vi "Node - Read Imported Channels.vi"(8 "error in (no error)":errorcluster, 10 "Node Name":string, 11 "Compiled.Settings In":T1) -> (0 "error out":errorcluster, 2 "Local Channels Table out":string[][](array[string]), 3 "Compiled.Settings Out":T1)   [LabVIEW 2016, in "PXImc Custom Device System Explorer.lvlib"]
uses:
  PXImc Custom Device System Explorer.lvlib
  Shared/Compiled.Settings.ctl
  <vilib>/NI Veristand/VeriStand Data/Byte Buffer/Byte Buffer.lvclass
  PXImc Router/Controls/Target Type.ctl
  PXImc Router/Controls/Router - Configuration.ctl
  PXImc Router/Controls/Router/Node Block R-W Properties.ctl
  PXImc Router/Controls/Router/Block Properties.ctl
  PXImc Router/Controls/Router/Router - PXImc Properties.ctl
  PXImc Router/Controls/Router/Router - PXImc Card Properties.ctl
  PXImc Router/Controls/Node Data.ctl
  PXImc Router/Controls/Node/Node - PXImc Parameters.ctl
  PXImc Router/Controls/Node/Node - Writer Data.ctl
  PXImc Router/Controls/Node/Node Ch Properties.ctl
  PXImc Router/Controls/Data Type.ctl
  PXImc Router/Controls/Node/Node - Readers Data.ctl
  PXImc Router/Controls/Node/Node - Reader Data.ctl
  <vilib>/Utility/file.llb/Read Delimited Spreadsheet (string).vi
  PXImc Router/PXImc Router.lvlib
  Shared/PXImc Custom Device Shared.lvlib
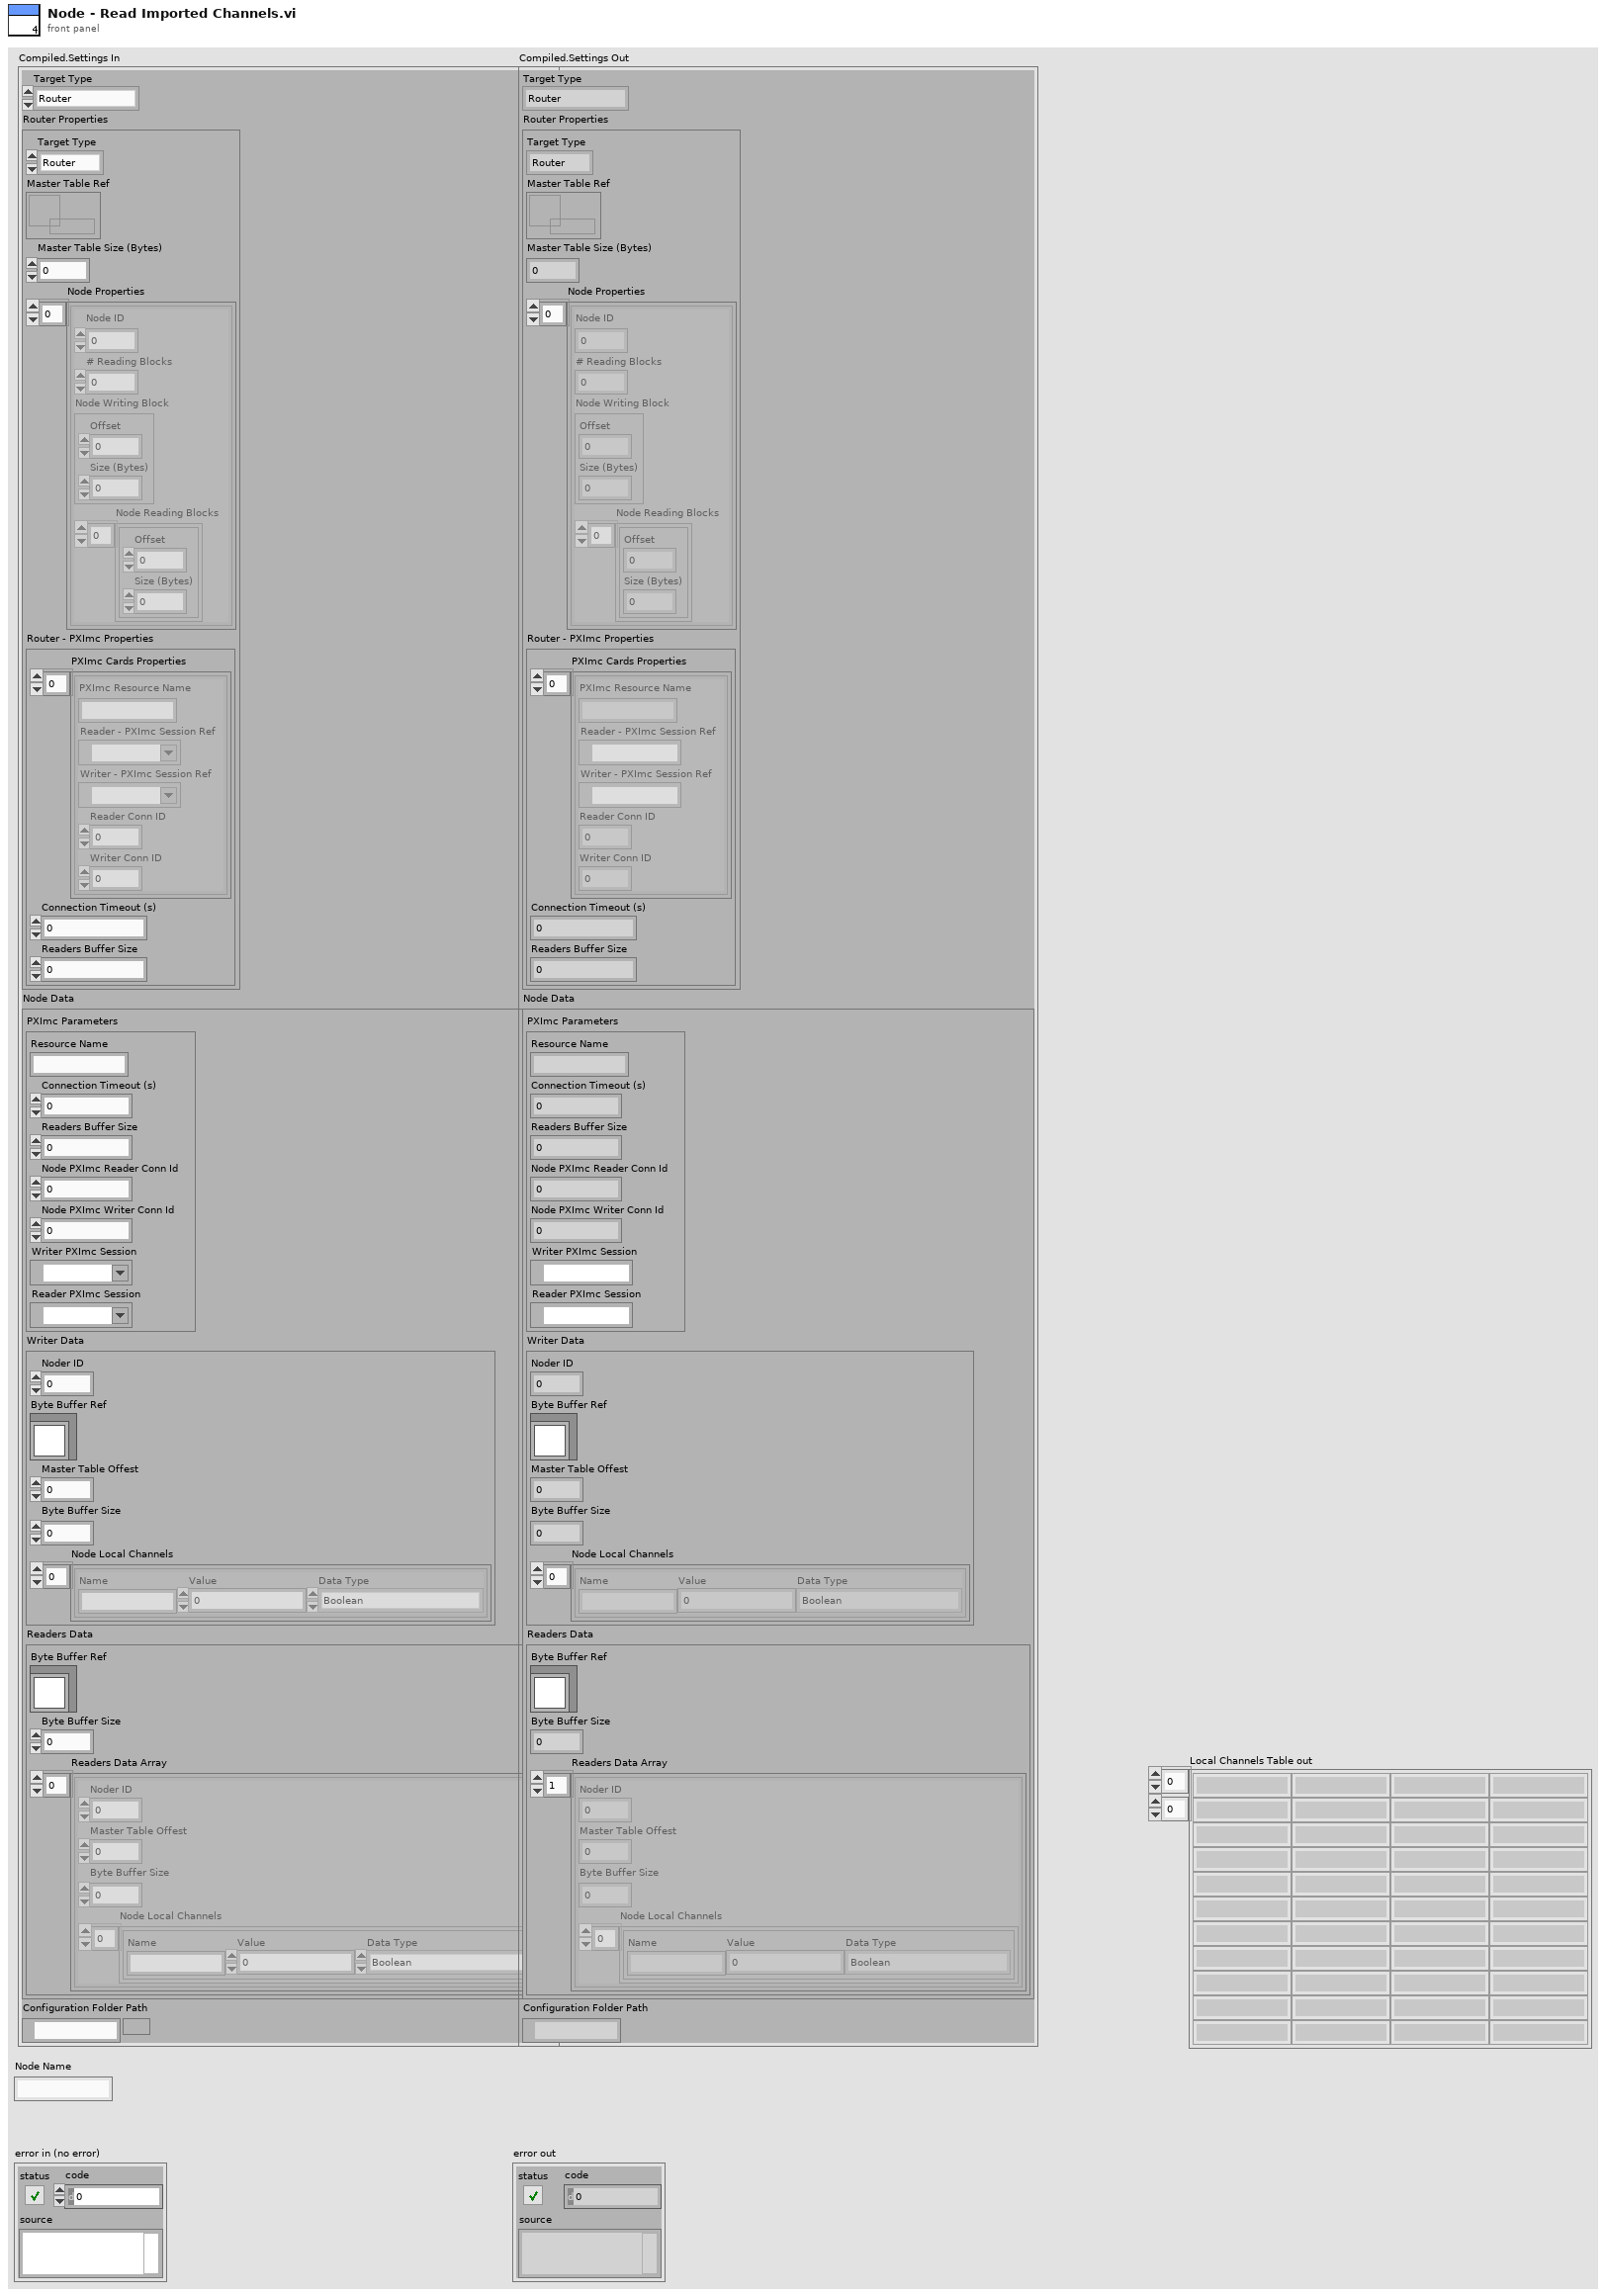
[diagram p1: front panel]
types:
  T1 = typedef "PXImc Custom Device Shared.lvlib/Compiled.Settings.ctl" = cluster{"Target Type":T2, "Router Properties":T3, "Node Data":T8, "Configuration Folder Path":path}
  T2 = typedef "PXImc Router.lvlib/Target Type.ctl" = enum16{"Router", "Node"}
  T3 = typedef "PXImc Router.lvlib/Router - Configuration.ctl" = cluster{"Target Type":T2, "Master Table Ref":refnum<data-value>, "Master Table Size (Bytes)":u32, "Node Properties":T4[], "Router - PXImc Properties":T6}
  T4 = typedef "PXImc Router.lvlib/Node Block R-W Properties.ctl" = cluster{"Node ID":u32, "# Reading Blocks":u32, "Node Writing Block":T5, "Node Reading Blocks":T5[]}
  T5 = typedef "PXImc Router.lvlib/Block Properties.ctl" = cluster{"Offset":u32, "Size (Bytes)":u32}
  T6 = typedef "PXImc Router.lvlib/Router - PXImc Properties.ctl" = cluster{"PXImc Cards Properties":T7[], "Connection Timeout (s)":dbl, "Readers Buffer Size":u64}
  T7 = typedef "PXImc Router.lvlib/Router - PXImc Card Properties.ctl" = cluster{"PXImc Resource Name":string, "Reader - PXImc Session Ref":refnum<k21>, "Writer - PXImc Session Ref":refnum<k21>, "Reader Conn ID":u16, "Writer Conn ID":u16}
  T8 = typedef "PXImc Router.lvlib/Node Data.ctl" = cluster{"PXImc Parameters":T9, "Writer Data":T10, "Readers Data":T13}
  T9 = typedef "PXImc Router.lvlib/Node - PXImc Parameters.ctl" = cluster{"Resource Name":string, "Connection Timeout (s)":dbl, "Readers Buffer Size":u64, "Node PXImc Reader Conn Id":u16, "Node PXImc Writer Conn Id":u16, "Writer PXImc Session":refnum<k21>, "Reader PXImc Session":refnum<k21>}
  T10 = typedef "PXImc Router.lvlib/Node - Writer Data.ctl" = cluster{"Noder ID":u32, "Byte Buffer Ref":refnum<class "Byte Buffer.lvclass">, "Master Table Offest":u32, "Byte Buffer Size":u32, "Node Local Channels":T11[]}
  T11 = typedef "PXImc Router.lvlib/Node Ch Properties.ctl" = cluster{"Name":string, "Value":dbl, "Data Type":T12}
  T12 = typedef "PXImc Router.lvlib/Data Type.ctl" = enum16{"Boolean", "SGL", "DBL", "I8", "I16", "I32", "I64", "U8", "U16", "U32", "U64"}
  T13 = typedef "PXImc Router.lvlib/Node - Readers Data.ctl" = cluster{"Byte Buffer Ref":refnum<class "Byte Buffer.lvclass">, "Byte Buffer Size":u64, "Readers Data Array":T14[]}
  T14 = typedef "PXImc Router.lvlib/Node - Reader Data.ctl" = cluster{"Noder ID":u32, "Master Table Offest":u32, "Byte Buffer Size":u64, "Node Local Channels":T11[]}
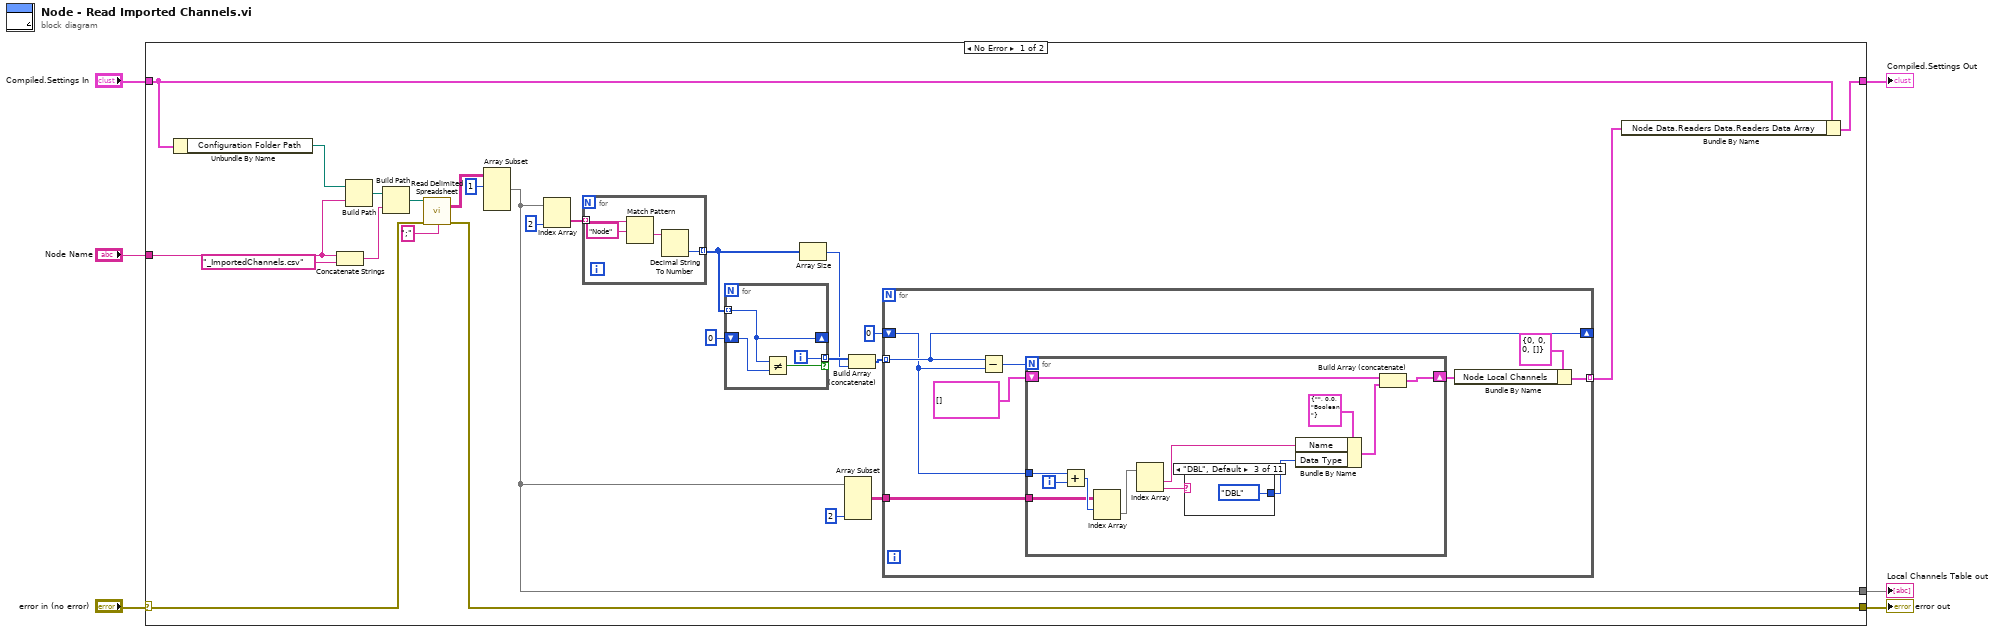
[diagram p0: block diagram]
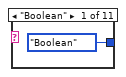
[diagram p2: hidden frame]
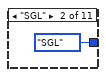
[diagram p3: hidden frame]
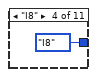
[diagram p4: hidden frame]
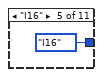
[diagram p5: hidden frame]
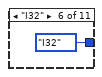
[diagram p6: hidden frame]
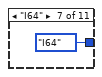
[diagram p7: hidden frame]
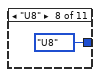
[diagram p8: hidden frame]
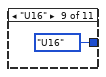
[diagram p9: hidden frame]
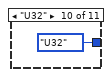
[diagram p10: hidden frame]
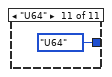
[diagram p11: hidden frame]
diagram:
  n1 = case shown="No Error" "error in (no error)" {
    selector: "error in (no error)" -> [w20 w71]
    tunnel: "Compiled.Settings In" -> [w27 w72]
    tunnel: [w28 w72] -> w5
    tunnel: [w19 w71] -> w3
    tunnel: "Node Name" -> [w25 _]
    tunnel: [w16 _] -> w1
    frame No Error {
      n2 = Unbundle By Name(w27) -> ("Configuration Folder Path"=w26:path)
      n3 = Concatenate Strings(w25, "_ImportedChannels.csv" ("name or relative path")) -> (w23:string)
      n4 = Build Path(base path=w26, name or relative path=w25) -> (appended path=w31:path)
      n5 = Build Path(base path=w31, name or relative path=w23) -> (appended path=w30:path)
      n6 = call-poly <vilib>:"Read Delimited Spreadsheet.vi"("file path (dialog if empty)"=w30, "error in (no error)"=w20, "delimiter (\\t)"=";" ("delimiter (\\t)")) -> ("all rows"=w22:string[][], "error out"=w19:errorcluster)  [unwired: 7 in, 4 out]
      n7 = Array Subset(array=w22, index (row)=1 ("index")) -> (w16:string[][])  [unwired: 3 in]
      n8 = Index Array(array=w16, index (col)=2 ("disabled index (col)")) -> (element=w17:string[])  [unwired: 1 in]
      n9 = for {
        tunnel: w17 -> [w70] mode=indexing
        tunnel: [w67] -> w9 mode=indexing
        n10 = Match Pattern(string=w70, regular expression="Node") -> (after substring=w68:string)  [unwired: 1 in, 3 out]
        n11 = Decimal String To Number(string=w68) -> (number=w67:i32)  [unwired: 2 in, 1 out]
      }
      n12 = for {
        tunnel: w9 -> [w65] mode=indexing
        shift-right: [w65] -> _
        shift-left: 0 -> [w66]
        tunnel: [w63] -> w10 mode=indexing if=w64
        i -> [w63]
        n13 = Not Equal?(x=w65, y=w66) -> (x != y?=w64:bool)
      }
      n14 = Array Size(array=w9) -> (size(s)=w7:i32)
      n15 = Array Subset(array=w16, length (col)=2 ("length")) -> (w14:string[][])  [unwired: 3 in]
      n16 = Build Array (concatenate)(w10, w7) -> (w8:i32[])
      n17 = for {
        tunnel: w8 -> [w34] mode=indexing
        tunnel: [w35] -> w13 mode=indexing
        shift-right: [w34] -> _
        shift-left: 0 -> [w33]
        tunnel: w14 -> [w39]
        n18 = Subtract(x=w34, y=w33) -> (x-y=w32:i32)
        n19 = for {
          N: w32 -> [_]
          tunnel: w33 -> [w41]
          shift-right: [w42] -> w36
          shift-left: T11[] [] ("Node Local Channels") -> [w43]
          tunnel: w39 -> [w46]
          i -> [w40]
          n20 = Add(x=w41, y=w40) -> (x+y=w47:i32)
          n21 = Index Array(array=w46, index (row)=w47) -> (element=w50:string[])  [unwired: 1 in]
          n22 = Index Array(array=w50) -> (element #1=w49:string, element #2=w48:string)  [unwired: 2 in]
          n23 = case shown="\"DBL\", Default" w48 {
            tunnel: [Data_Type."Boolean" ("Data Type") Data_Type."SGL" ("Data Type") Data_Type."DBL" ("Data Type") Data_Type."I8" ("Data Type") Data_Type."I16" ("Data Type") Data_Type."I32" ("Data Type") Data_Type."I64" ("Data Type") Data_Type."U8" ("Data Type") Data_Type."U16" ("Data Type") Data_Type."U32" ("Data Type") Data_Type."U64" ("Data Type")] -> w51
            frame "Boolean" {
            }
            frame "SGL" {
            }
            frame "DBL", Default {
            }
            frame "I8" {
            }
            frame "I16" {
            }
            frame "I32" {
            }
            frame "I64" {
            }
            frame "U8" {
            }
            frame "U16" {
            }
            frame "U32" {
            }
            frame "U64" {
            }
          }
          n24 = Bundle By Name(cluster=T11 {"Name"="", "Value"=0.0, "Data Type"=enum."Boolean"} ("Node Ch Properties"), "Name"=w49, "Data Type"=w51) -> (w44:T11)
          n25 = Build Array (concatenate)(w43, w44) -> (w42:T11[])
        }
        n26 = Bundle By Name(cluster=T14 {"Noder ID"=0, "Master Table Offest"=0, "Byte Buffer Size"=0, "Node Local Channels"=[]} ("Reader Data"), "Node Local Channels"=w36) -> (w35:T14)
      }
      n27 = Bundle By Name(cluster=w27, "Node Data.Readers Data.Readers Data Array"=w13) -> (w28:T1)
    }
    frame Error {
    }
  }
  "Compiled.Settings Out" <- w5
  "error out" <- w3
  "Local Channels Table out" <- w1
